vi "test_libssh2_channel_forward_listen.vi"() -> ()   [LabVIEW 2017, in "integration_tests.lvlib"]
uses:
  integration_tests.lvlib
  libssh2/libssh2_channel_forward_listen_ex.vi
  support/support.lvlib
  libssh2/libssh2.lvlib
  <vilib>/PNR/Transparent Assertions/Transparent Assertions/Transparent Assertions.lvlib
panel:
  out "error out":errorcluster
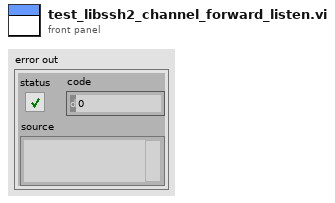
[diagram p1: front panel]
types:
  T1 = typedef "libssh2.lvlib/Session Refnum.ctl" = refnum<k1>
  T2 = typedef "libssh2.lvlib/Listener Refnum.ctl" = refnum<k1>
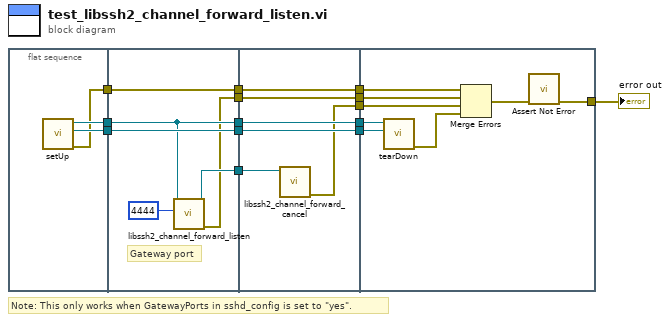
[diagram p0: block diagram]
diagram:
  # "Note: This only works when GatewayPorts in sshd_config is set to \"yes\"."
  n1 = flat-sequence {
    tunnel: [w17] -> w14
    tunnel: [w16] -> w13
    tunnel: [w15] -> w12
    tunnel: w14 -> [w21]
    tunnel: w13 -> [w23]
    tunnel: [w21] -> w6
    tunnel: [w23] -> w5
    tunnel: w12 -> [w22]
    tunnel: [w22] -> w4
    tunnel: [w20] -> w3
    tunnel: [w18] -> w2
    tunnel: w6 -> [w29]
    tunnel: [w29] -> w10
    tunnel: w5 -> [w28]
    tunnel: [w28] -> w9
    tunnel: w4 -> [w27]
    tunnel: [w27] -> w8
    tunnel: [w25] -> w7
    tunnel: w3 -> [w26]
    tunnel: w2 -> [w24]
    tunnel: [w24] -> w1
    tunnel: w10 -> [w37]
    tunnel: w9 -> [w36]
    tunnel: [w35] -> w11
    tunnel: w8 -> [w33]
    tunnel: w7 -> [w31]
    tunnel: w1 -> [w30]
    frame #0 {
      n2 = call "setUp.vi"() -> ("error out"=w15:errorcluster, "connection ID"=w16:refnum<k5>, "session"=w17:T1)  [unwired: 9 in]
    }
    frame #1 {
      # "Gateway port"
      n3 = call "libssh2_channel_forward_listen.vi"("port in"=4444, "session"=w21) -> ("error out"=w18:errorcluster, "listener"=w20:T2)  [unwired: 7 in, 1 out]
    }
    frame #2 {
      n4 = call "libssh2_channel_forward_cancel.vi"("listener"=w26) -> ("error out"=w25:errorcluster)  [unwired: 10 in]
    }
    frame #3 {
      n5 = call "tearDown.vi"("connection ID"=w36, "session"=w37) -> ("error out"=w34:errorcluster)  [unwired: 9 in]
      n6 = Merge Errors(w33, w30, w31, w34) -> (w32:errorcluster)
      n7 = call <vilib>:"Assert Not Error.vi"("error in (no error)"=w32) -> ("error out"=w35:errorcluster)  [unwired: 10 in]
    }
  }
  "error out" <- w11
